vi "Configure Hardware.vi"(8 "error in (no error)":errorcluster, 11 "Hardware Configuration In":T1={"Accel-ai0"=FALSE, "Maximum Input"=0.0, "Minimum Input"=0.0, "Sample Rate"=0.0, "Number of Samples"=8192, "Accel-ai1"=FALSE, "DAQmx Task"="", "Low Pass Filter"={"Upper Cutoff"=350.0, "Lower Cutoff"=350.0, "Order"=350}} {"Low Pass Filter"."Order" min=0 max=10 step=1}) -> (0 "error out":errorcluster, 3 "Hardware Configuration Out":T1={"Accel-ai0"=FALSE, "Maximum Input"=0.0, "Minimum Input"=0.0, "Sample Rate"=0.0, "Number of Samples"=0, "Accel-ai1"=FALSE, "DAQmx Task"="", "Low Pass Filter"={"Upper Cutoff"=350.0, "Lower Cutoff"=350.0, "Order"=350}} {"Low Pass Filter"."Order" min=0 max=10 step=1})   [LabVIEW 2022 SP3, in "Acquisition.lvlib"]
doc: "Configure the hardware."
uses:
  Acquisition.lvlib
  FiniteMeasurement-DAQmx/controls/Hardware Configuration.ctl
  AcquisitionFilter.ctl
  <vilib>/DAQmx/configure/timing.llb/DAQmx Timing (Sample Clock).vi
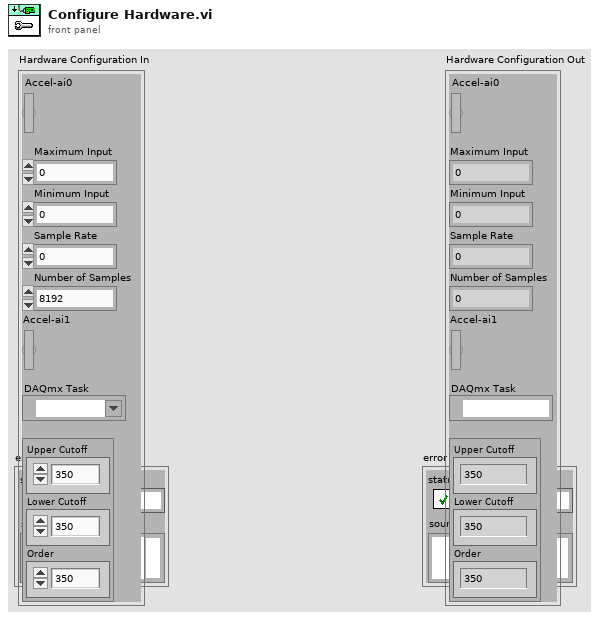
[diagram p1: front panel]
types:
  T1 = typedef "Acquisition.lvlib/Hardware Configuration.ctl" = cluster{"Accel-ai0":bool, "Maximum Input":dbl, "Minimum Input":dbl, "Sample Rate":dbl, "Number of Samples":i32, "Accel-ai1":bool, "DAQmx Task":refnum<k21>, "Low Pass Filter":T2}
  T2 = typedef "AcquisitionFilter.ctl" = cluster{"Upper Cutoff":dbl, "Lower Cutoff":dbl, "Order":i32}
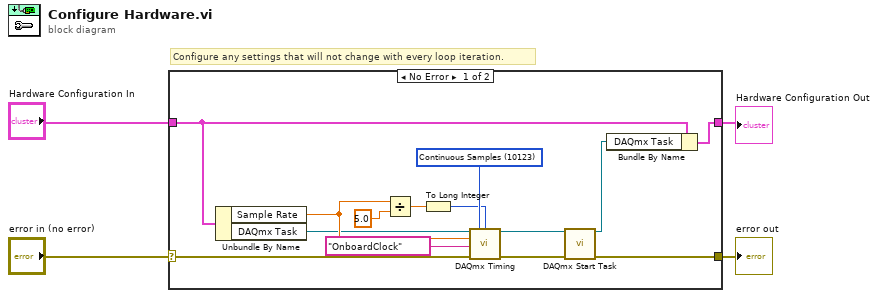
[diagram p0: block diagram]
diagram:
  # "Configure any settings that will not change with every loop iteration."
  n1 = case shown="No Error" "error in (no error)" {
    selector: "error in (no error)" -> [w12 w19]
    tunnel: [w13 w19] -> w3
    tunnel: "Hardware Configuration In" -> [w8 w20]
    tunnel: [w6 w20] -> w1
    frame No Error {
      w18 = 10123 items=["Finite Samples"=10178, "Continuous Samples"=10123, "Hardware Timed Single Point"=12522] ("sample mode")
      n2 = Unbundle By Name(w8) -> ("Sample Rate"=w11:dbl, "DAQmx Task"=w10:refnum<k21>)
      n3 = Divide(x=w11, y=5.0) -> (x/y=w16:dbl)
      n4 = To Long Integer(number=w16) -> (32bit integer=w9:i32)
      n5 = call-poly <vilib>:"DAQmx Timing.vi"("task/channels in"=w10, "sample mode"=w18, "samples per channel"=w9, "rate"=w11, "source"=tag "OnboardClock", "error in"=w12) -> ("task out"=w14:refnum<k21>, "error out"=w15:errorcluster)  [unwired: 8 in]
      n6 = call <vilib>:"DAQmx Start Task.vi"("task/channels in"=w14, "error in"=w15) -> ("task out"=w7:refnum<k21>, "error out"=w13:errorcluster)  [unwired: 12 in]
      n7 = Bundle By Name(cluster=w8, "DAQmx Task"=w7) -> (w6:T1)
    }
    frame Error {
    }
  }
  "error out" <- w3
  "Hardware Configuration Out" <- w1
